vi "Read Label.vi"(11 "Properties in":refnum<class "Properties.lvclass">) -> (2 "Test Label":string, 3 "Properties out":refnum<class "Properties.lvclass">)   [LabVIEW 2013, in "Caraya.lvlib" / "Properties.lvclass"]
uses:
  Properties.lvclass
  Properties.lvclass/Properties.ctl
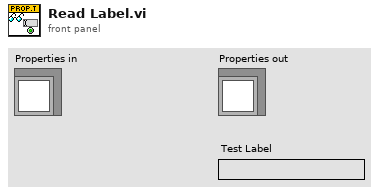
[diagram p1: front panel]
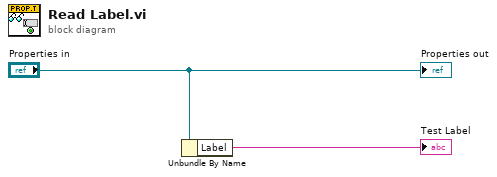
[diagram p0: block diagram]
diagram:
  n1 = Unbundle By Name("Properties in") -> ("Label"=→"Test Label":string)
  "Properties out" <- "Properties in"
